vi "Read Log Session.vi"(8 "error in":errorcluster, 11 "Ex Nested in":refnum<class "SuperActor.lvclass">) -> (0 "error out":errorcluster, 2 "Session Handle":T1, 3 "Ex Nested out":refnum<class "SuperActor.lvclass">)   [LabVIEW 2016, in "SuperActor.lvlib" / "SuperActor.lvclass"]
uses:
  SuperActor.lvclass
  Session APIs/_Session Fwk/Typedefs/Session Handle.ctl
  Session APIs/_Session Fwk/Session - Root.lvclass
  SuperActor.lvclass/SuperActor.ctl
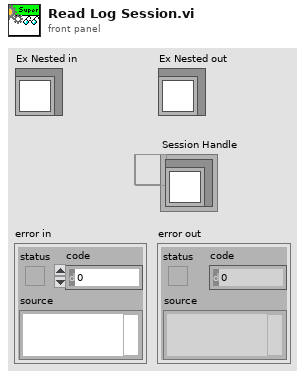
[diagram p1: front panel]
types:
  T1 = typedef "Session - Root.lvclass/Session Handle.ctl" = refnum<data-value>
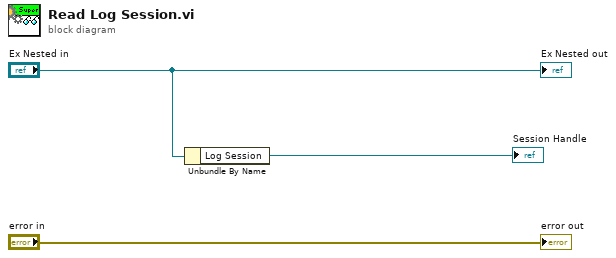
[diagram p0: block diagram]
diagram:
  n1 = Unbundle By Name("Ex Nested in") -> ("Log Session"=→"Session Handle":T1)
  "error out" <- "error in"
  "Ex Nested out" <- "Ex Nested in"
